vi "sub5choice.vi"(8 "error in":errorcluster, 10 "Detector Start Pin":u8, 11 "Arduino Resource":T1={"VISA resource"="", "Board Type"=enum."Uno", "Connection Type"=enum."USB / Serial", "Bytes Per Packet (15)"=15}) -> (0 "error out":errorcluster, 2 "Numeric":dbl, 3 "Arduino Resource 2":T1={"VISA resource"="", "Board Type"=enum."Uno", "Connection Type"=enum."USB / Serial", "Bytes Per Packet (15)"=15})   [LabVIEW 2016]
uses:
  <vilib>/LabVIEW Interface for Arduino/Type Defs/Arduino Resource.ctl
  <vilib>/LabVIEW Interface for Arduino/Type Defs/Board Type.ctl
  <vilib>/LabVIEW Interface for Arduino/LabVIEW Interface for Arduino.lvlib
panel:
  out "Boolean":bool
  out "Boolean 2":bool
  out "Boolean 3":bool
  out "Boolean 4":bool
  out "Boolean 5":bool
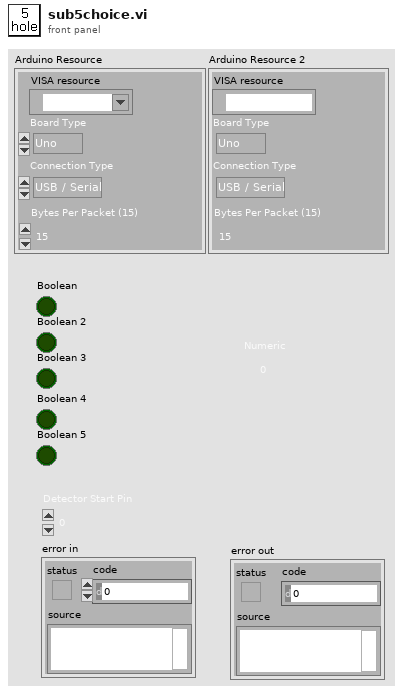
[diagram p1: front panel]
types:
  T1 = typedef "LabVIEW Interface for Arduino.lvlib/Arduino Resource.ctl" = cluster{"VISA resource":refnum<visa-resource-name>, "Board Type":T2, "Connection Type":enum8{"USB / Serial"}, "Bytes Per Packet (15)":u8}
  T2 = typedef "LabVIEW Interface for Arduino.lvlib/Board Type.ctl" = enum16{"Uno", "Dimuelanove w/Atmega 328", "Mega 2560"}
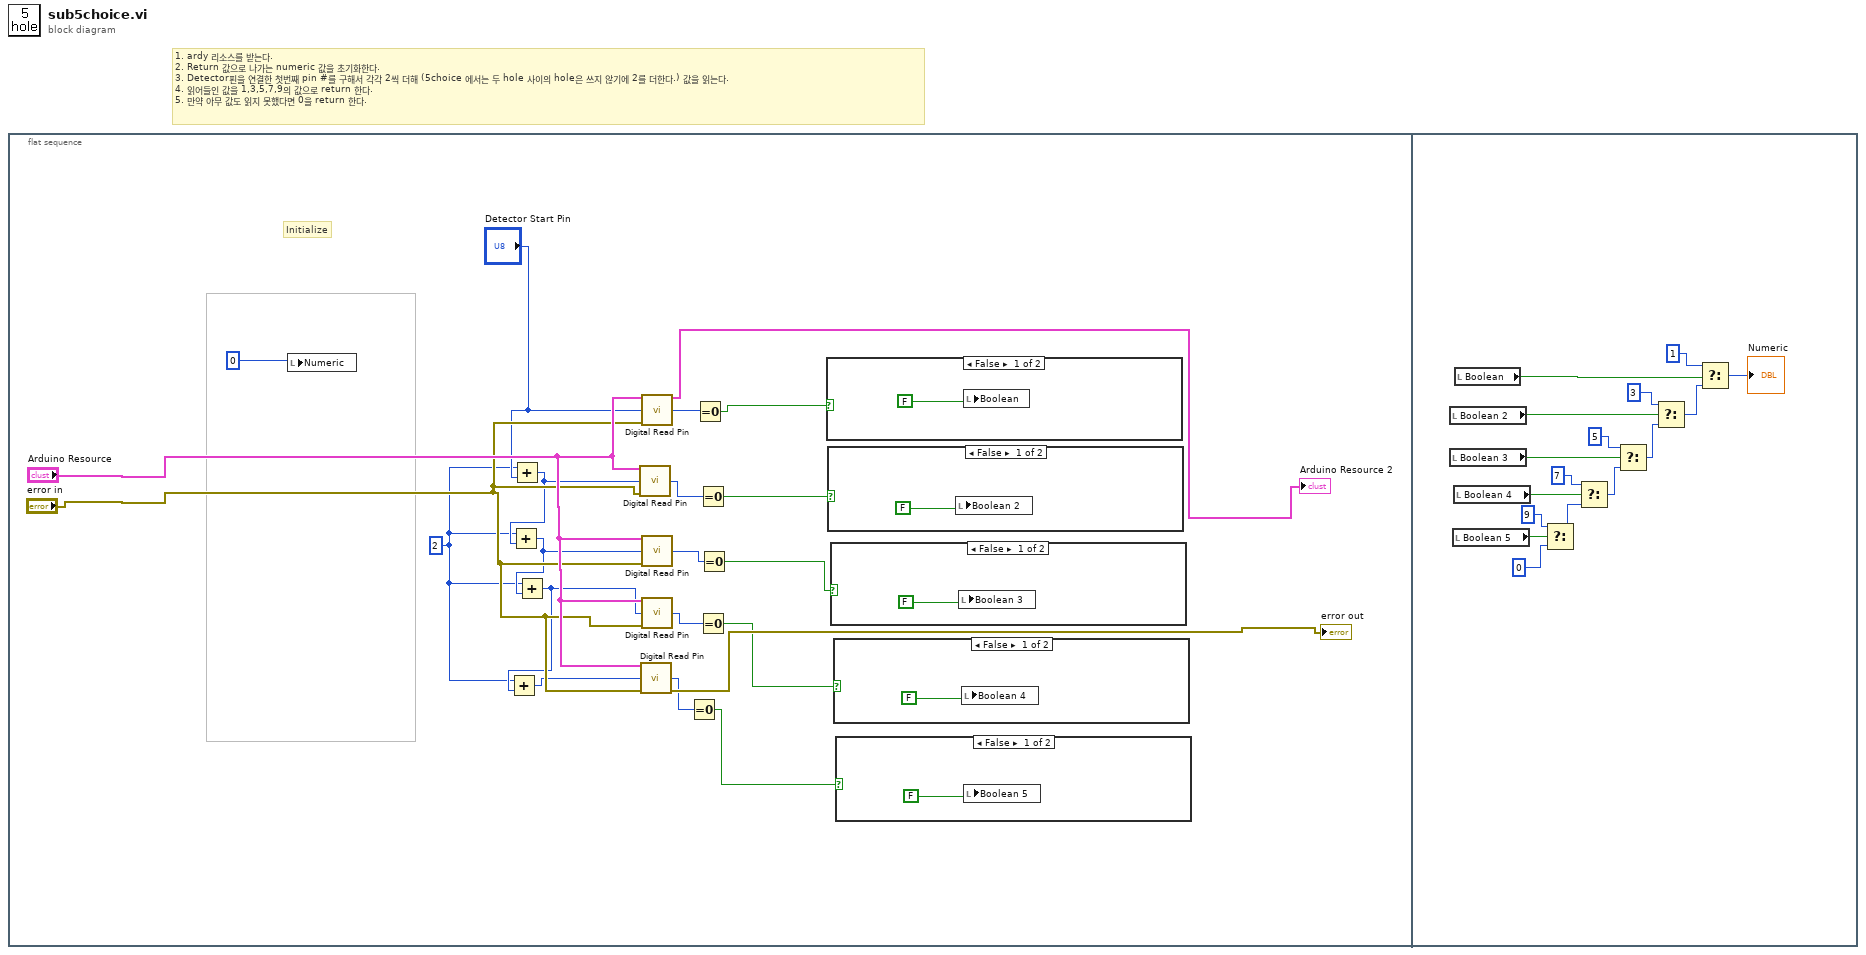
[diagram p0: block diagram]
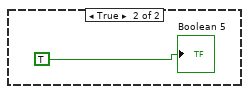
[diagram p2: hidden frame]
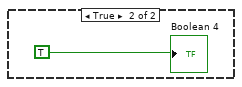
[diagram p3: hidden frame]
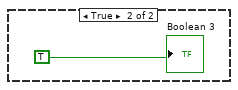
[diagram p4: hidden frame]
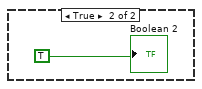
[diagram p5: hidden frame]
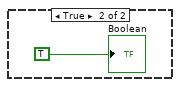
[diagram p6: hidden frame]
diagram:
  # "1. ardy 리소스를 받는다. \n2. Return 값으로 나가는 numeric 값을 초기화한다.\n3. Detector핀을 연결한 첫번째 pin #를 구해서 각각 2씩 더해 (5choice 에서는 두 hole 사이의 hole은 쓰지 않기에 2를 더한다.) 값을 읽는다.\n4. 읽어들인 값을 1,3,5,7,9의 값으로 return 한다. \n5. 만약 아무 값도 읽지 못했다면 0을 return 한다."
  n1 = flat-sequence {
    frame #0 {
      w1 = 2
      # "Initialize"
      n2 = local write "Numeric"(0) -> ()
      n3 = Add(x=w1, y="Detector Start Pin") -> (x+y=w5:i32)
      n4 = Add(x=w1, y=w5) -> (x+y=w4:i32)
      n5 = Add(x=w1, y=w4) -> (x+y=w3:i32)
      n6 = Add(x=w1, y=w3) -> (x+y=w2:i32)
      n7 = call <vilib>:"Digital Read Pin.vi"("Arduino Resource"="Arduino Resource", "Digital I/O Pin (0)"=w5, "error in"="error in") -> ("Value"=w10:u8)  [unwired: 10 in, 2 out]
      n8 = call <vilib>:"Digital Read Pin.vi"("Arduino Resource"="Arduino Resource", "Digital I/O Pin (0)"=w2, "error in"="error in") -> ("Value"=w7:u8, "error out"=→"error out":errorcluster)  [unwired: 10 in, 1 out]
      n9 = call <vilib>:"Digital Read Pin.vi"("Arduino Resource"="Arduino Resource", "Digital I/O Pin (0)"="Detector Start Pin", "error in"="error in") -> ("Arduino Resource"=→"Arduino Resource 2":T1, "Value"=w11:u8)  [unwired: 10 in, 1 out]
      n10 = call <vilib>:"Digital Read Pin.vi"("Arduino Resource"="Arduino Resource", "Digital I/O Pin (0)"=w4, "error in"="error in") -> ("Value"=w9:u8)  [unwired: 10 in, 2 out]
      n11 = call <vilib>:"Digital Read Pin.vi"("Arduino Resource"="Arduino Resource", "Digital I/O Pin (0)"=w3, "error in"="error in") -> ("Value"=w8:u8)  [unwired: 10 in, 2 out]
      n12 = Equal To 0?(x=w7) -> (x = 0?=w12:bool)
      n13 = Equal To 0?(x=w11) -> (x = 0?=w16:bool)
      n14 = Equal To 0?(x=w10) -> (x = 0?=w15:bool)
      n15 = Equal To 0?(x=w8) -> (x = 0?=w13:bool)
      n16 = Equal To 0?(x=w9) -> (x = 0?=w14:bool)
      n17 = case shown="False" w16 {
        frame False {
          n18 = local write "Boolean"(FALSE) -> ()
        }
        frame True {
          "Boolean" <- TRUE
        }
      }
      n19 = case shown="False" w15 {
        frame False {
          n20 = local write "Boolean 2"(FALSE) -> ()
        }
        frame True {
          "Boolean 2" <- TRUE
        }
      }
      n21 = case shown="False" w14 {
        frame False {
          n22 = local write "Boolean 3"(FALSE) -> ()
        }
        frame True {
          "Boolean 3" <- TRUE
        }
      }
      n23 = case shown="False" w13 {
        frame False {
          n24 = local write "Boolean 4"(FALSE) -> ()
        }
        frame True {
          "Boolean 4" <- TRUE
        }
      }
      n25 = case shown="False" w12 {
        frame False {
          n26 = local write "Boolean 5"(FALSE) -> ()
        }
        frame True {
          "Boolean 5" <- TRUE
        }
      }
    }
    frame #1 {
      n27 = local read "Boolean 2"() -> (w45:bool)
      n28 = local read "Boolean 3"() -> (w44:bool)
      n29 = local read "Boolean 5"() -> (w39:bool)
      n30 = local read "Boolean 4"() -> (w41:bool)
      n31 = local read "Boolean"() -> (w47:bool)
      n32 = Select(t=9, s=w39, f=0) -> (s? t:f=w40:i32)
      n33 = Select(t=7, s=w41, f=w40) -> (s? t:f=w42:i32)
      n34 = Select(t=5, s=w44, f=w42) -> (s? t:f=w43:i32)
      n35 = Select(t=3, s=w45, f=w43) -> (s? t:f=w46:i32)
      n36 = Select(t=1, s=w47, f=w46) -> (s? t:f=→"Numeric":i32)
    }
  }
